vi "DtCreateAinRawChan.vi"(1 "Channel Type":i32(ring)=100 items=["SingleEnded"=100, "Differential"=101], 2 "Range Min":dbl=-10.0, 3 "Range Max":dbl=10.0, 5 "Board Name":string, 7 "Channel":string="Ain 0", 9 "Element":u32, 11 "error in (no error)":errorcluster) -> (4 "Task out":i32, 8 "Actual Number of Channels":u32, 15 "error out":errorcluster)   [LabVIEW 2022 SP3]
doc: "Creates one or more virtual analog input channels to measure raw counts. \n\nIf your device supports streaming digital inputs, counter/timers, and/or quadrature decoder inputs through the analog input subsystem, this VI also creates one or more virtual channels for the digital input ports, counter/timer channels, and/or quadrature decoder channels."
uses:
  DtLvLink.lvlib
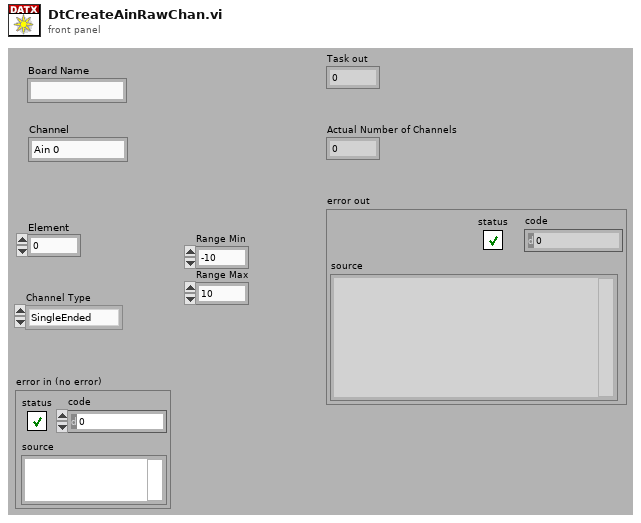
[diagram p1: front panel]
types:
  T1 = enum32{"AnalogInput", "AnalogOutput", "DigitalInput", "DigitalOutput", "Quadrature", "CounterTimer"}
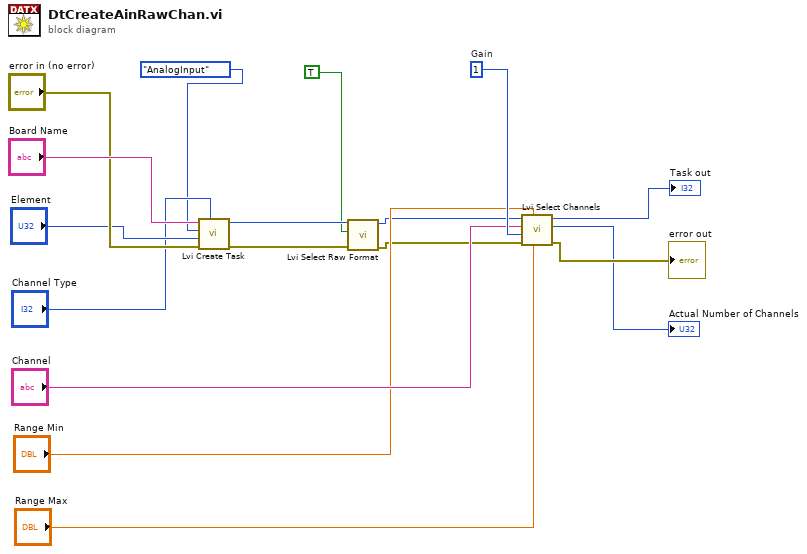
[diagram p0: block diagram]
diagram:
  w17 = u32 1  # Gain
  n1 = call "Lvi Create Task.vi"("SEorDiff"="Channel Type", "error in (no error)"="error in (no error)", "SubSysIndex"="Element", "ChanType"=T1."AnalogInput", "BoardName"="Board Name") -> ("error out"=w5:errorcluster, "TaskRef"=w7:i32)  [unwired: 4 in, 1 out]
  n2 = call "Lvi Select Raw Format.vi"("error in (no error)"=w5, "RawFormat"=TRUE ("Boolean RawFormat"), "TaskRef"=w7) -> ("error out"=w4:errorcluster, "TaskRef out"=w6:i32)  [unwired: 6 in, 1 out]
  n3 = call "Lvi Select Channels.vi"("MaxRange"="Range Max", "MinRange"="Range Min", "error in (no error)"=w4, "Gain"=w17, "ChanListStr"="Channel", "TaskRef"=w6) -> ("error out"=→"error out":errorcluster, "ActualNumChannels"=→"Actual Number of Channels":u32, "TaskRef out"=→"Task out":i32)  [unwired: 2 in, 1 out]
